vi "Inverse Filter.vi"(0 "Noise in":refnum<class "Noise.lvclass">, 5 "Level in":refnum<class "Level.lvclass">, 7 "Fs (Hz)":dbl, 9 "Npts":i32, 11 "error in (no error)":errorcluster) -> (4 "Noise out":refnum<class "Noise.lvclass">, 8 "noise":dbl[](array[numeric]), 10 "reference":dbl, 15 "error out":errorcluster)   [LabVIEW 2020, in "Noise.lvclass"]
uses:
  Noise.lvclass
  Level/Level.lvclass
  Noise.lvclass/Noise.ctl
  Level/Level.lvclass/Level.ctl
  Utility VIs/Math VIs/Linear to dB (scalar).vi
  Utility VIs/Math VIs/FFT x(t) to dB,Degrees (1D).vi
  <vilib>/Analysis/NI_AALBase.lvlib
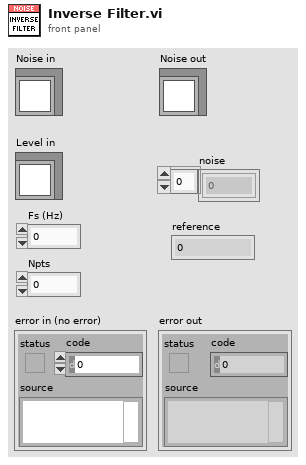
[diagram p1: front panel]
types:
  T1 = cluster{"Freq (Hz)":dbl[], "Mag (dB SPL)":dbl[], "Phase (deg)":dbl[]}
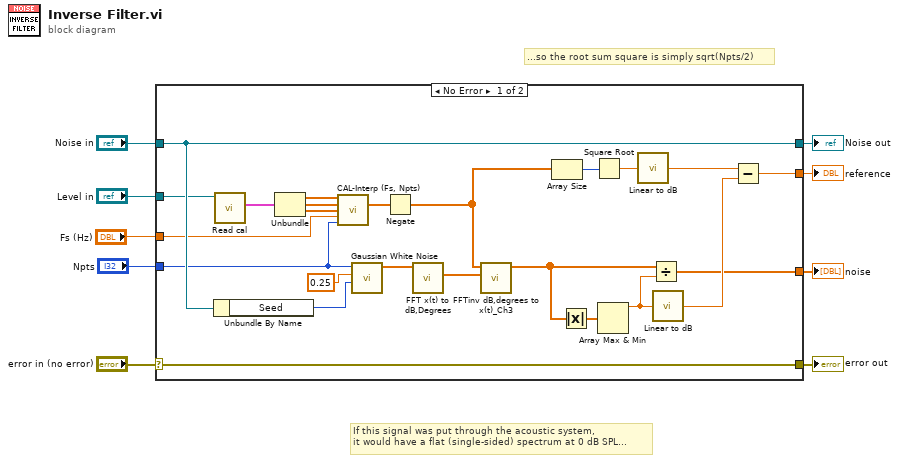
[diagram p0: block diagram]
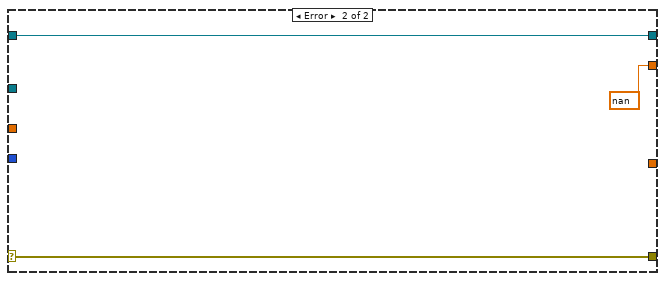
[diagram p2: hidden frame]
diagram:
  # "...so the root sum square is simply sqrt(Npts/2)"
  # "If this signal was put through the acoustic system,\nit would have a flat (single-sided) spectrum at 0 dB SPL..."
  n1 = case shown="No Error" "error in (no error)" {
    selector: "error in (no error)" -> [w33 w36]
    tunnel: [w33 w36] -> w8
    tunnel: [w31 w35] -> w6
    tunnel: "Noise in" -> [w31 w35]
    tunnel: "Level in" -> [w27 _]
    tunnel: "Npts" -> [w12 _]
    tunnel: "Fs (Hz)" -> [w13 _]
    tunnel: [w16 nan] -> w2
    tunnel: [w18 _] -> w1
    frame No Error {
      n2 = Unbundle By Name(w31) -> ("Seed"=w30:i32)
      n3 = call "Read cal.vi"("Level in"=w27) -> ("cal"=w26:T1)  [unwired: 8 in, 2 out]
      n4 = Unbundle(w26) -> ("Freq (Hz)"=w25:dbl[], "Mag (dB SPL)"=w24:dbl[], "Phase (deg)"=w23:dbl[])
      n5 = call "CAL-Interp (Fs, Npts).vi"("Frequency (Hz)"=w25, "Magnitude (dB)"=w24, "Phase (degrees)"=w23, "Fs (Hz)"=w13, "Npts"=w12) -> ("Interp Magnitude (dB)"=w14:dbl[])  [unwired: 7 in, 3 out]
      n6 = call <vilib>:"Gaussian White Noise.vi"("seed"=w30, "standard deviation"=0.25, "samples"=w12) -> ("Gaussian noise pattern"=w29:dbl[])  [unwired: 7 in, 1 out]
      n7 = Negate(x=w14) -> (-x=w10:dbl[])
      n8 = call-poly "FFT x(t) to dB,Degrees.vi"("X"=w29) -> ("+Freq Phase of FFT (degrees)"=w28:dbl[])  [unwired: 8 in, 2 out]
      n9 = call "FFTinv dB,degrees to x(t)_Ch3.vi"("+Freq Phase of FFT (degrees)"=w28, "+Freq. Mag of FFT (rms dB)"=w10) -> ("X(t)"=w15:dbl[])  [unwired: 8 in, 1 out]
      n10 = Array Size(array=w10) -> (size(s)=w11:i32)
      n11 = Absolute Value(x=w15) -> (abs(x)=w22:dbl[])
      n12 = Square Root(x=w11) -> (sqrt(x)=w17:dbl)
      n13 = Array Max & Min(array=w22) -> (max value=w20:dbl)  [unwired: 3 out]
      n14 = call-poly "Linear to dB.vi"("Linear"=w17) -> ("dB"=w19:dbl)
      n15 = Divide(x=w15, y=w20) -> (x/y=w18:dbl[])
      n16 = call-poly "Linear to dB.vi"("Linear"=w20) -> ("dB"=w21:dbl)
      n17 = Subtract(x=w19, y=w21) -> (x-y=w16:dbl)
    }
    frame Error {
    }
  }
  "error out" <- w8
  "Noise out" <- w6
  "reference" <- w2
  "noise" <- w1
